vi "dfd_Build 2-band Analysis Bank and Synthesis Bank from TFs.vi"(6 "fs":dbl=1.0, 7 "processing method":T1, 8 "error in (no error)":errorcluster, 10 "F 0":dbl[](array[numeric]), 11 "H 0":dbl[](array[numeric])) -> (0 "error out":errorcluster, 2 "synthesis bank":T2 {"mBank_Type" items=["Uniform", "Non-Uniform"]; "mBank_Filters"."mMRate_SumWl" min=1 max=32 step=1; "mBank_Filters"."mMRate_InputIwl" min=1 max=32 step=1; "mBank_Filters"."mMRate_GainWl" min=1 max=32 step=1; "mBank_Filters"."mMRate_OutputWl" min=1 max=32 step=1; "mBank_Filters"."mMRate_InputWl" min=1 max=32 step=1; "mBank_Filters"."mMRate_CoefWl" min=1 max=32 step=1; "mBank_Filters"."mMRate_Mode" items=["Default"=-1, "No Rate Change"=0, "Interpolation"=1, "Decimation"=2, "Interpolated"=3, "Rational"=4]}, 3 "analysis bank":T2 {"mBank_Type" items=["Uniform", "Non-Uniform"]; "mBank_Filters"."mMRate_SumWl" min=1 max=32 step=1; "mBank_Filters"."mMRate_InputIwl" min=1 max=32 step=1; "mBank_Filters"."mMRate_GainWl" min=1 max=32 step=1; "mBank_Filters"."mMRate_OutputWl" min=1 max=32 step=1; "mBank_Filters"."mMRate_InputWl" min=1 max=32 step=1; "mBank_Filters"."mMRate_CoefWl" min=1 max=32 step=1; "mBank_Filters"."mMRate_Mode" items=["Default"=-1, "No Rate Change"=0, "Interpolation"=1, "Decimation"=2, "Interpolated"=3, "Rational"=4]})   [LabVIEW 2017, in "NI_DigFilter_FilterBank.lvlib"]
uses:
  <vilib>/addons/Digital Filter Design/NI_DigFilter_FilterBank.lvlib
  <vilib>/addons/Digital Filter Design/FilterBank.llb/Object/DFD Bank Obj.ctl
  <vilib>/addons/Digital Filter Design/_Objects.llb/DFD Multirate Filter Obj.ctl
  <vilib>/addons/Digital Filter Design/_Objects.llb/DFD Multirate Mode.ctl
  <vilib>/addons/Digital Filter Design/_Objects.llb/DFD Coef Norm Type.ctl
  <vilib>/addons/Digital Filter Design/_Objects.llb/DFD Round-off Mode.ctl
  <vilib>/addons/Digital Filter Design/_Objects.llb/DFD FXP MRate Multiply Mode.ctl
  <vilib>/addons/Digital Filter Design/FilterBank.llb/Object/DFD Filter Bank Processing Method.ctl
  <vilib>/addons/Digital Filter Design/FilterBank.llb/Object/DFD Filter Bank Type.ctl
  <vilib>/addons/Digital Filter Design/NI_DigFilterLicensed.lvlib
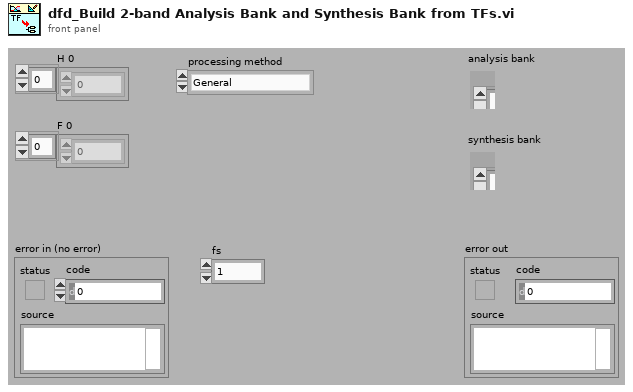
[diagram p1: front panel]
types:
  T1 = typedef "NI_DigFilter_FilterBank.lvlib/DFD Filter Bank Processing Method.ctl" = enum16{"General", "2-Band QMF Lattice", "Cosine-Modulated"}
  T2 = typedef "NI_DigFilter_FilterBank.lvlib/DFD Bank Obj.ctl" = cluster{"mBank_Filters":T3[], " mBank_#Bands":i32, "mBank_ProcMethod":T1, "mBank_Coeffs":dbl[], "mBank_Gain":dbl, "mBank_Type":T8}
  T3 = typedef "NI_DigFilterLicensed.lvlib/DFD Multirate Filter Obj.ctl" = cluster{"mMRate_Structure":enum16{"CIC", "FIR", "IIR", "Lattice"}, "mMRate_Mode":T4, "mMRate_Factor":i32, "mMRate_FIRParams":cluster{"mMRate_FIR_H":dbl[], "mMRate_FIR_IsNyquist?":bool, "mMRate_FIR_IsSymmetric?":bool}, "mMRate_CICParams":cluster{"mMRate_CIC_#Stage":i32, "mMRate_CIC_Lag":i32, "mMRate_CIC_Type":enum16{"Lowpass", "Highpass"}}, "mMRate_Order":i32, "mMRate_Version":string, "mMRate_Comments":string, "mMRate_RationalFactor":cluster{"mMRate_L":i32, "mMRate_M":i32}, "mMRate_Fs":dbl, "mMRate_Quantized?":bool, "mMRate_QFilterGain":dbl, "mMRate_CoefWl":i16, "mMRate_Scaling":cluster{"mMRate_ScaleByPowerOf2?":bool, "mMRate_ScaleType":T5}, "mMRate_InputWl":i16, "mMRate_OutputWl":i16, "mMRate_OutputMode":T6, "mMRate_MultMode":T7, "mMRate_BitPruning":bool, "mMRate_GainWl":i16, "mMRate_OutputFwl":i16, "mMRate_SumIwl":i16, "mMRate_InputIwl ":i16, "mMRate_SumWl":i16, "mMRate_CoefIwl":i16}
  T4 = typedef "NI_DigFilterLicensed.lvlib/DFD Multirate Mode.ctl" = i16
  T5 = typedef "NI_DigFilterLicensed.lvlib/DFD Coef Norm Type.ctl" = enum16{"No Norm", "Time Domain 1-Norm", "Time Domain 2-Norm", "Time Domain Inf-Norm"}
  T6 = typedef "NI_DigFilterLicensed.lvlib/DFD Round-off Mode.ctl" = enum16{"Nearest", "Truncation"}
  T7 = typedef "NI_DigFilterLicensed.lvlib/DFD FXP MRate Multiply Mode.ctl" = enum16{"Truncated", "Full"}
  T8 = typedef "NI_DigFilter_FilterBank.lvlib/DFD Filter Bank Type.ctl" = u16
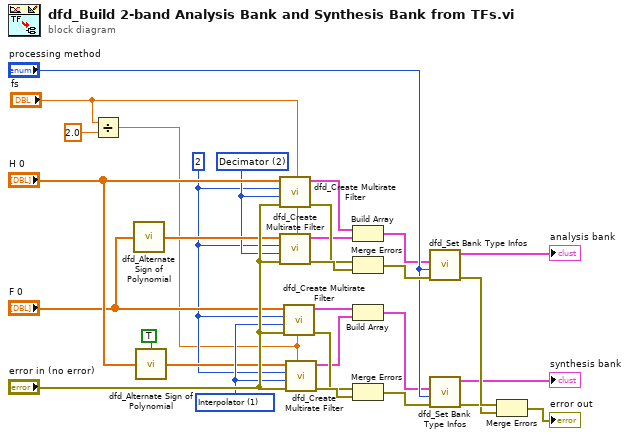
[diagram p0: block diagram]
diagram:
  w18 = T4 2 items=["Default"=-1, "Normal"=0, "Interpolator"=1, "Decimator"=2, "Interpolated"=3] ("mode")
  w17 = T4 1 items=["Default"=-1, "Normal"=0, "Interpolator"=1, "Decimator"=2, "Interpolated"=3] ("mode")
  w8 = 2 ("factor")
  n1 = Divide(x="fs", y=2.0) -> (x/y=w1:dbl)
  n2 = call <vilib>:"dfd_Alternate Sign of Polynomial.vi"("polynomial in"="F 0") -> ("polynomial out"=w19:dbl[])  [unwired: 1 in]
  n3 = call <vilib>:"dfd_Alternate Sign of Polynomial.vi"("polynomial in"="H 0", "even? (F)"=TRUE ("(-h)?")) -> ("polynomial out"=w16:dbl[])
  n4 = call <vilib>:"dfd_Create Multirate Filter.vi"("fs"="fs", "error in (no error)"="error in (no error)", "mode"=w18, "factor"=w8, "h (n)"="H 0") -> ("error out"=w24:errorcluster, "multirate filter out"=w12:T3)  [unwired: 5 in]
  n5 = call <vilib>:"dfd_Create Multirate Filter.vi"("fs"="fs", "error in (no error)"="error in (no error)", "mode"=w18, "factor"=w8, "h (n)"=w19) -> ("error out"=w29:errorcluster, "multirate filter out"=w11:T3)  [unwired: 5 in]
  n6 = call <vilib>:"dfd_Create Multirate Filter.vi"("fs"=w1, "error in (no error)"="error in (no error)", "mode"=w17, "factor"=w8, "h (n)"="F 0") -> ("error out"=w26:errorcluster, "multirate filter out"=w10:T3)  [unwired: 5 in]
  n7 = call <vilib>:"dfd_Create Multirate Filter.vi"("fs"=w1, "error in (no error)"="error in (no error)", "mode"=w17, "factor"=w8, "h (n)"=w16) -> ("error out"=w27:errorcluster, "multirate filter out"=w9:T3)  [unwired: 5 in]
  n8 = Build Array(w12, w11) -> (w13:T3[])
  n9 = Merge Errors(w24, w29) -> (w25:errorcluster)
  n10 = Build Array(w10, w9) -> (w14:T3[])
  n11 = Merge Errors(w26, w27) -> (w28:errorcluster)
  n12 = call <vilib>:"dfd_Set Bank Type Infos.vi"("error in (no error)"=w25, "processing method"="processing method", "subband filters"=w13) -> ("error out"=w6:errorcluster, "bank out"=→"analysis bank":T2)  [unwired: 7 in]
  n13 = call <vilib>:"dfd_Set Bank Type Infos.vi"("error in (no error)"=w28, "processing method"="processing method", "subband filters"=w14) -> ("error out"=w4:errorcluster, "bank out"=→"synthesis bank":T2)  [unwired: 7 in]
  n14 = Merge Errors(w6, w4) -> (→"error out":errorcluster)
